vi "inputOneEntry.vi"(8 "inputError":errorcluster, 10 "file path (dialog if empty)":path=path "G:/Document/랩타임측정시스템/Program/CommonResource/EVEntry.txt") -> (0 "outputError":errorcluster, 1 "StopButtonOutput":bool, 2 "OKButtonOutput":bool, 3 "CurrentData":T1)   [LabVIEW 2020]
uses:
  <vilib>/Utility/file.llb/Read Delimited Spreadsheet (string).vi
panel:
  in  "Input Entry":i32
  in  "Stop Button":bool
  in  "OK Button":bool
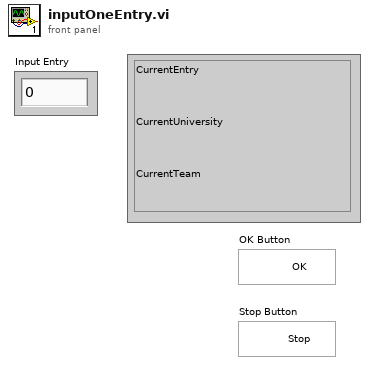
[diagram p1: front panel]
types:
  T1 = cluster{"CurrentEntry":string, "CurrentUniversity":string, "CurrentTeam":string}
  T2 = enum16{"open", "replace", "create", "open or create", "replace or create", "replace or create with confirmation"}
  T3 = cluster{"CurrentEntry":string, "CurrentUniv":string, "CurrentTeam":string}
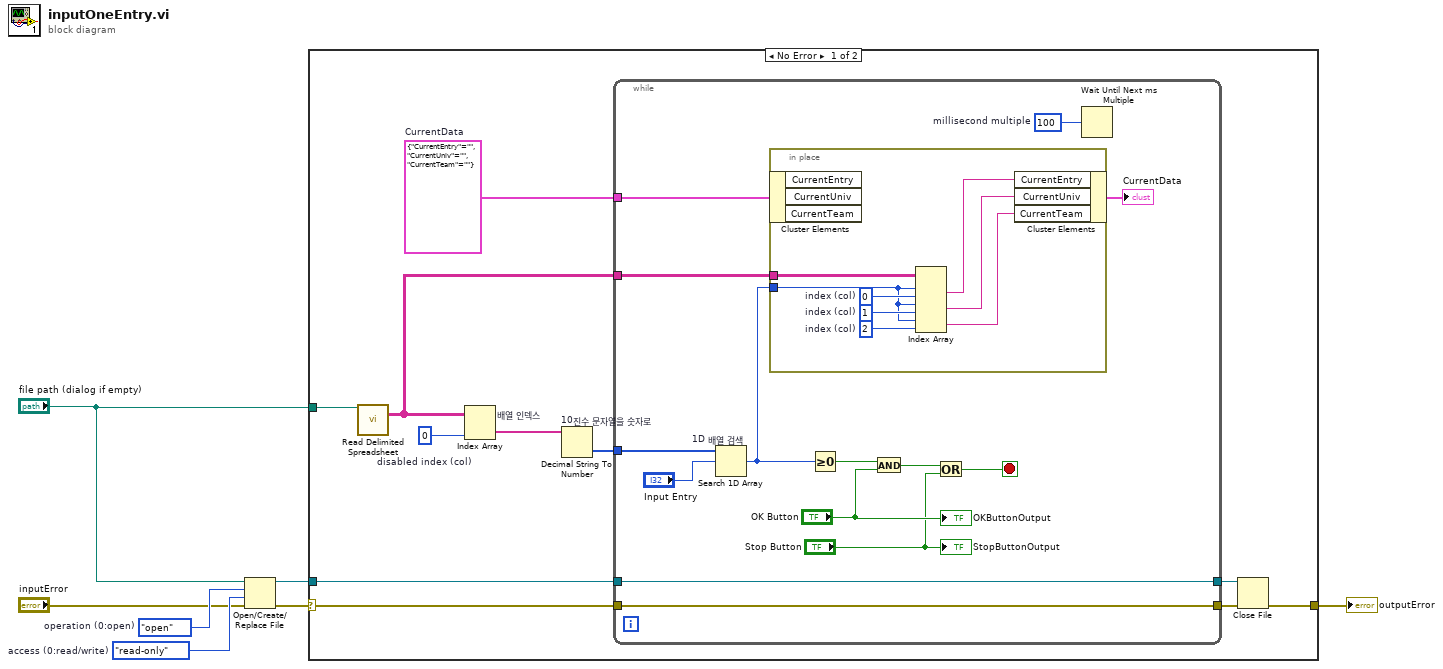
[diagram p0: block diagram]
diagram:
  w2 = enum16{"read/write", "read-only", "write-only"}."read-only"  # access (0:read/write)
  w4 = T2."open"  # operation (0:open)
  n1 = Open/Create/Replace File(file path (use dialog)="file path (dialog if empty)", error in="inputError", operation (0:open)=w4, access (0:read/write)=w2) -> (refnum out=w3:refnum<file>, error out=w7:errorcluster)  [unwired: 2 in, 1 out]
  n2 = case shown="No Error" w7 {
    selector: w7 -> [w8 w41]
    tunnel: [w12 w41] -> w6
    tunnel: "file path (dialog if empty)" -> [w17 _]
    tunnel: w3 -> [w10 _]
    frame No Error {
      w13 = 0  # disabled index (col)
      w15 = T3 {"CurrentEntry"="", "CurrentUniv"="", "CurrentTeam"=""}  # CurrentData
      n3 = call-poly <vilib>:"Read Delimited Spreadsheet.vi"("file path (dialog if empty)"=w17) -> ("all rows"=w14:string[][])  [unwired: 9 in, 5 out]
      n4 = Index Array "배열 인덱스"(array=w14, index (col)=w13) -> (element=w18:string[])  [unwired: 1 in]
      n5 = Decimal String To Number "10진수 문자열을 숫자로"(string=w18) -> (number=w16:i32[])  [unwired: 2 in, 1 out]
      n6 = while {
        tunnel: w16 -> [w27]
        tunnel: w14 -> [w26]
        tunnel: w15 -> [w22]
        tunnel: [w24] -> w11
        tunnel: w10 -> [w24]
        tunnel: [w23] -> w9
        tunnel: w8 -> [w23]
        stop <- w29 stop-if-true
        w19 = u32 100  # millisecond multiple
        n7 = Search 1D Array "1D 배열 검색"(1D array=w27, element="Input Entry") -> (index of element=w20:i32)  [unwired: 1 in]
        n8 = in-place {
          in-place-border: w26 -> [w40]
          in-place-border: w20 -> [w33]
          w34 = 2  # index (col)
          w35 = 1  # index (col)
          w36 = 0  # index (col)
          n9 = in-place-cluster #1(w22) -> ()  [unwired: 3 out]
          n10 = Index Array "Index Array"(array=w40, index (row) #1=w33, index (col) #1=w36, index (row) #2=w33, index (col) #2=w35, index (row) #3=w33, index (col) #3=w34) -> (element #1=w39:string, element #2=w38:string, element #3=w37:string)
          n11 = in-place-cluster #1("CurrentEntry"=w39, "CurrentUniv"=w38, "CurrentTeam"=w37) -> (→"CurrentData":T3)
        }
        n12 = Greater Or Equal To 0?(x=w20) -> (x >= 0?=w32:bool)
        n13 = And(x=w32, y="OK Button") -> (x .and. y?=w31:bool)
        n14 = Or(x=w31, y="Stop Button") -> (x .or. y?=w29:bool)
        n15 = Wait Until Next ms Multiple(millisecond multiple=w19) -> ()  [unwired: 1 out]
        "OKButtonOutput" <- "OK Button"
        "StopButtonOutput" <- "Stop Button"
      }
      n16 = Close File(refnum=w11, error in=w9) -> (error out=w12:errorcluster)  [unwired: 1 out]
    }
    frame Error {
    }
  }
  "outputError" <- w6
